vi "test controller.vi"() -> ()   [LabVIEW 2024, in "Lock-in module.lvlib"]
uses:
  Lock-in module.lvlib
  Messenger service/MessengerLib.lvlib
  Messenger service/Data types/Mailbox address.ctl
  ctl/MFLI_command enum.ctl
  ctl/MFLI_message for module.ctl
  <instrlib>/Zurich Instruments LabOne/Public/ziTypeHandle.ctl
  <instrlib>/Zurich Instruments LabOne/Zurich Instruments LabOne.lvlib
  <instrlib>/Zurich Instruments LabOne/Public/Data/ziTypeDemodSampleSingle.ctl
  ctl/MFLI parameters.ctl
  ctl/Mode.ctl
  ctl/ACQ info.ctl
panel:
  out "error out":errorcluster
  out "ignored error":errorcluster
  out "data":errorcluster
  out "Waveform Graph 3":dbl[](graph)
  out "LockIn info":T1
  out "data 2":T2={"Timestamps (ticks)"=0, "X (Vrms)"=nan, "Y (Vrms)"=nan, "Osc Phase (deg)"=nan, "Freq (Hz)"=nan, "DIO"=0, "AuxIn0 (V)"=nan, "AuxIn1 (V)"=nan, "Trigger"=0}
  out "Lock-in handle":T3 {"Handle" format="0x%08x"; "Conn" format="0x%08x"}
  out "Parameters out":T4={"Filter order"=1.0, "Time constant [ms]"=1.0, "F_Mod [kHz]"=0.0, "Amp_Mod [mV]"=0.0, "Enable output"=0, "Phase [°]"=0.0} {"Enable output" items=["Disable", "Enable"]; "Filter order" min=1.0 step=1.0; "Time constant [ms]" min=1.0 max=9.0 step=1.0}
  out "Array":string[](array[string])
  out "Connected device":string
  in  "Device name":string="DEV4029"
  in  "ACQ parameters":T4={"Filter order"=1.0, "Time constant [ms]"=1.0, "F_Mod [kHz]"=0.0, "Amp_Mod [mV]"=0.0, "Enable output"=0, "Phase [°]"=0.0} {"Enable output" items=["Disable", "Enable"]; "F_Mod [kHz]" min=0.1 max=100.0; "Filter order" min=1.0 max=9.0 step=1.0; "Time constant [ms]" min=0.001 max=1000000000.0}
  in  "Stop Button":bool
  in  "Connect":bool
  in  "Update settings":bool
  in  "Record":bool
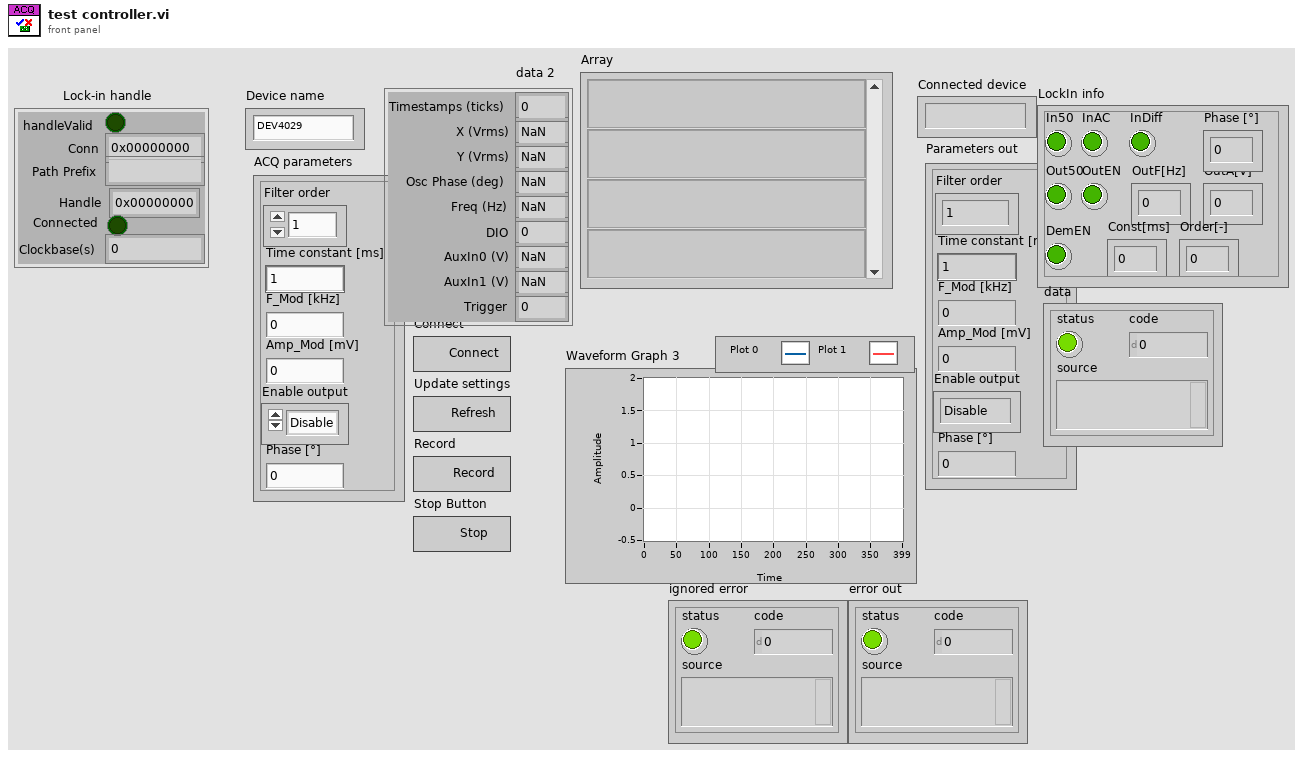
[diagram p1: front panel]
types:
  T1 = typedef "Lock-in module.lvlib/ACQ info.ctl" = cluster{"In50":bool, "InAC":bool, "InDiff":bool, "Out50":bool, "OutEN":bool, "OutF[Hz]":dbl, "OutA[V]":dbl, "DemEN":bool, "Const[ms]":dbl, "Order[-]":i32, "Phase [°]":dbl}
  T2 = typedef "Zurich Instruments LabOne.lvlib/ziTypeDemodSampleSingle.ctl" = cluster{"Timestamps (ticks)":u64, "X (Vrms)":dbl, "Y (Vrms)":dbl, "Osc Phase (deg)":dbl, "Freq (Hz)":dbl, "DIO":u32, "AuxIn0 (V)":dbl, "AuxIn1 (V)":dbl, "Trigger":u32}
  T3 = typedef "Zurich Instruments LabOne.lvlib/ziTypeHandle.ctl" = cluster{"handleValid":bool, "Conn":u64, "Path Prefix":string, "Handle":u64, "Connected":bool, "Clockbase(s)":dbl}
  T4 = typedef "Lock-in module.lvlib/MFLI parameters.ctl" = cluster{"Filter order":dbl, "Time constant [ms]":dbl, "F_Mod [kHz]":dbl, "Amp_Mod [mV]":dbl, "Enable output":u16, "Phase [°]":dbl}
  T5 = typedef "MessengerLib.lvlib/Mailbox address.ctl" = refnum<queue>
  T6 = typedef "MessengerLib.lvlib/Messenger referencies.ctl" = cluster{"TOP":refnum<queue>, "Instr_M":refnum<queue>, "Field_C":refnum<queue>, "Tmp_M":refnum<queue>, "Tmp_C":refnum<queue>, "Table_C":refnum<queue>, "MW_C":refnum<queue>, "Data_Aq":refnum<queue>, "Mod_M":refnum<queue>, "Field_M":refnum<queue>, "Pwr_M":refnum<queue>, "Angle_C":refnum<queue>, "Sample_C":refnum<queue>, "Reserved":refnum<queue>}
  T7 = typedef "Lock-in module.lvlib/MFLI_message for module.ctl" = cluster{"Command":T8, "Data":variant}
  T8 = typedef "Lock-in module.lvlib/MFLI_command enum.ctl" = enum16{"Initialize", "Update", "Set parameters", "Set module", "Set individual parameters", "Get point", "Get array", "Disconnect", "End", "Ignore"}
  T9 = typedef "Lock-in module.lvlib/Mode.ctl" = enum16{"None", "Point", "Scope", "Both", "DAQ"}
  T10 = typedef "MessengerLib.lvlib/MSG to TOP.ctl" = cluster{"Module":T11, "Response":string, "Data":variant, "Time":timestamp}
  T11 = typedef "Module name.ctl" = enum16{"Emty", "Magnet", "VTI", "Excitation", "Servo", "Acquisition", "Rotator", "Digitizer", "SMU2450", "Carousel", "Multimeter", "Tmp monitor", "Power monitor"}
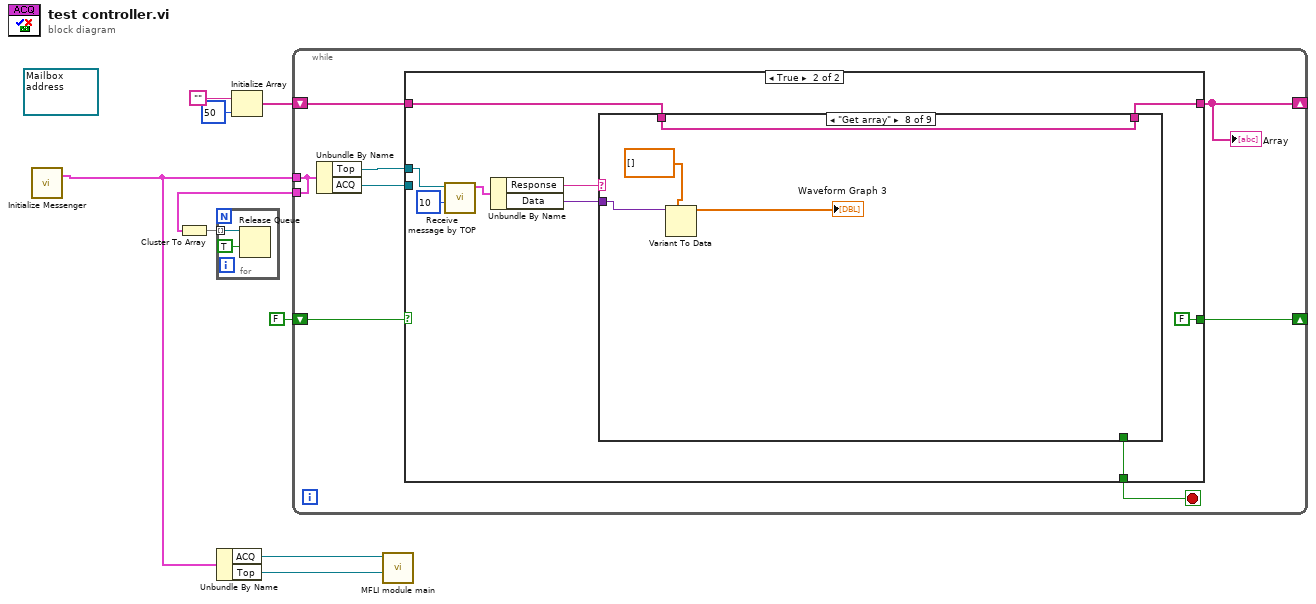
[diagram p0: block diagram]
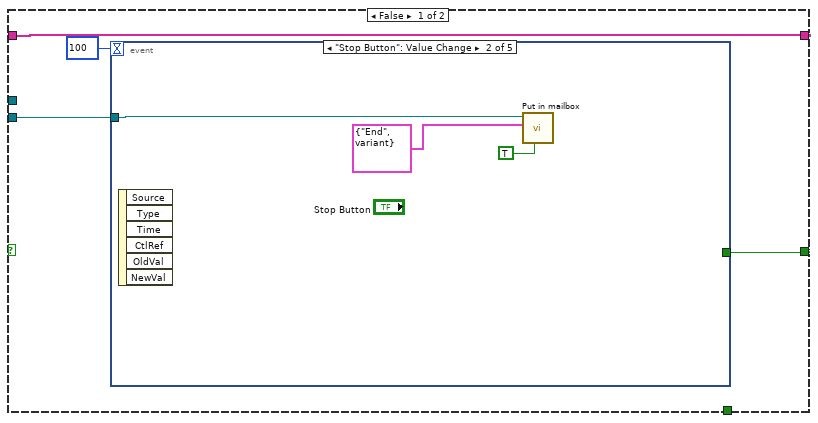
[diagram p2: hidden frame]
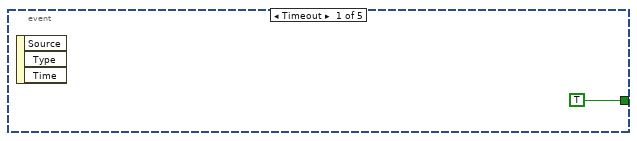
[diagram p3: hidden frame]
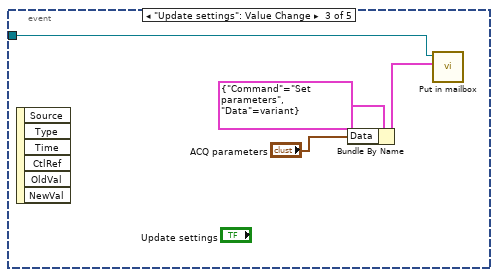
[diagram p4: hidden frame]
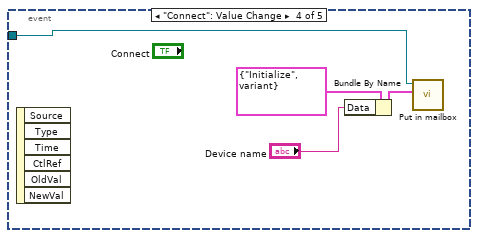
[diagram p5: hidden frame]
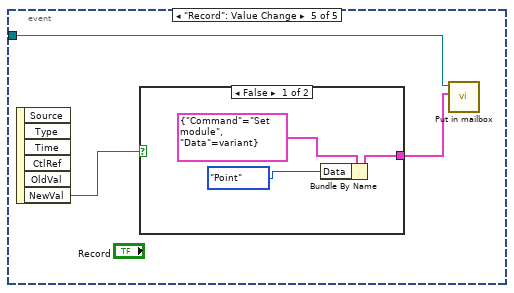
[diagram p6: hidden frame]
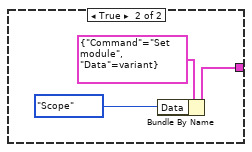
[diagram p7: hidden frame]
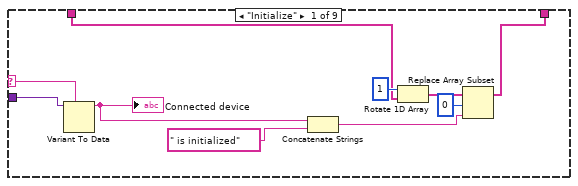
[diagram p8: hidden frame]
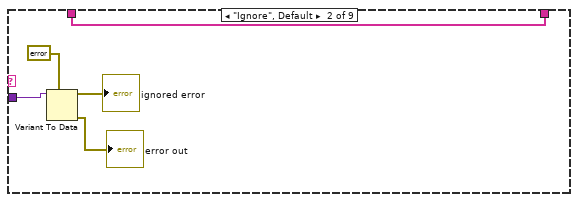
[diagram p9: hidden frame]
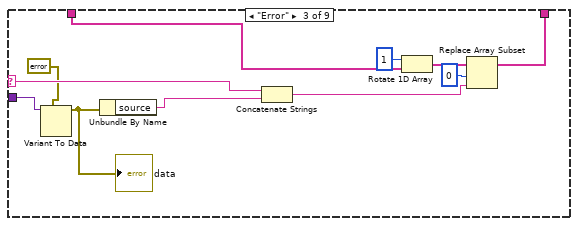
[diagram p10: hidden frame]
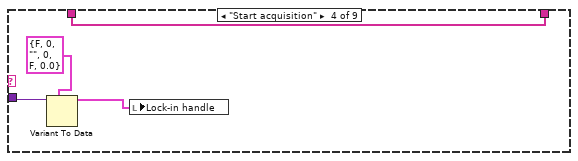
[diagram p11: hidden frame]
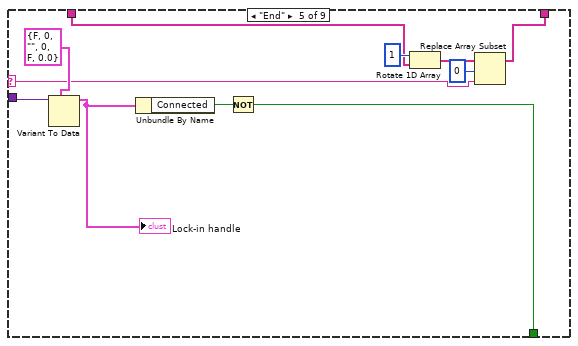
[diagram p12: hidden frame]
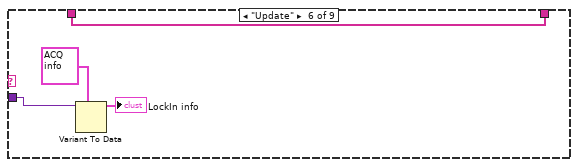
[diagram p13: hidden frame]
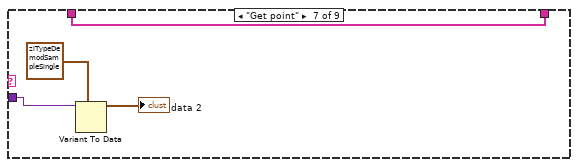
[diagram p14: hidden frame]
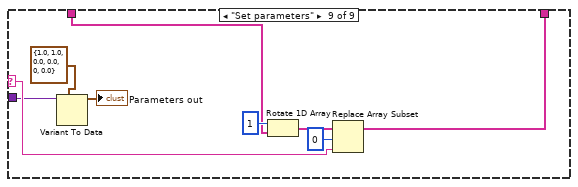
[diagram p15: hidden frame]
diagram:
  (unwired) T5 refnum ("Digitizer")
  n1 = call "Initialize Messenger.vi"() -> ("Referencies out"=w3:T6)  [unwired: 2 in, 1 out]
  n2 = Unbundle By Name(w3) -> ("ACQ"=w1:refnum<queue>, "Top"=w2:refnum<queue>)
  n3 = Initialize Array("", 50 ("dimension size")) -> (w4:string[])
  n4 = while {
    shift-right: [w16] -> _
    shift-left: FALSE -> [w17]
    tunnel: w3 -> [w12]
    tunnel: [w12] -> w8
    shift-right: [w10] -> _
    shift-left: w4 -> [w11]
    stop <- w15 stop-if-true
    n5 = Unbundle By Name(w12) -> ("Top"=w14:refnum<queue>, "ACQ"=w13:refnum<queue>)
    n6 = case shown="True" w17 {
      tunnel: [w20 FALSE] -> w16
      tunnel: w14 -> [_ w50]
      tunnel: w13 -> [w19 _]
      tunnel: [_ w46] -> w15
      tunnel: w11 -> [w18 w45]
      tunnel: [w18 w44] -> w10
      frame False {
        n7 = event shown="[1] \"Stop Button\": Value Change" {
          selector: _ -> [_ _ _ _ _]
          dyn-events: _ -> [_ _ _ _ _]
          timeout: 100 -> [_ _ _ _ _]
          tunnel: [TRUE _ _ _ _] -> w20
          tunnel: w19 -> [_ w25 w26 w32 w36]
          event Timeout {
            n8 = event-data() -> ()  [unwired: 1 in, 3 out]
          }
          event "Stop Button": Value Change {
            n9 = event-data() -> ()  [unwired: 1 in, 6 out]
            n10 = call "Put in mailbox.vi"("Priority? (F)"=TRUE, "Message"=T7 {"Command"=enum."End", "Data"=variant} ("MSG for  ACQ"), "Queue in"=w25) -> ()  [unwired: 6 in, 3 out]
          }
          event "Update settings": Value Change {
            n11 = event-data() -> ()  [unwired: 1 in, 6 out]
            n12 = Bundle By Name(cluster=T7 {"Command"=enum."Set parameters", "Data"=variant} ("MSG for  ACQ"), "Data"="ACQ parameters") -> (w28:T7)
            n13 = call "Put in mailbox.vi"("Message"=w28, "Queue in"=w26) -> ()  [unwired: 7 in, 3 out]
          }
          event "Connect": Value Change {
            n14 = event-data() -> ()  [unwired: 1 in, 6 out]
            n15 = Bundle By Name(cluster=T7 {"Command"=enum."Initialize", "Data"=variant} ("MSG for  ACQ"), "Data"="Device name") -> (w31:T7)
            n16 = call "Put in mailbox.vi"("Message"=w31, "Queue in"=w32) -> ()  [unwired: 7 in, 3 out]
          }
          event "Record": Value Change {
            n17 = event-data() -> ("NewVal"=w34:bool)  [unwired: 1 in, 5 out]
            n18 = case shown="False" w34 {
              tunnel: [w38 w41] -> w35
              frame False {
                n19 = Bundle By Name(cluster=T7 {"Command"=enum."Set module", "Data"=variant} ("MSG for  ACQ"), "Data"=Mode."Point" ("Mode")) -> (w38:T7)
              }
              frame True {
                n20 = Bundle By Name(cluster=T7 {"Command"=enum."Set module", "Data"=variant} ("MSG for  ACQ"), "Data"=Mode."Scope" ("Mode")) -> (w41:T7)
              }
            }
            n21 = call "Put in mailbox.vi"("Message"=w35, "Queue in"=w36) -> ()  [unwired: 7 in, 3 out]
          }
        }
      }
      frame True {
        n22 = call "Receive message by TOP.vi"("timeout (100)"=10 ("timeout (-1)"), "Mailbox in"=w50) -> ("MSG packet"=w49:T10)  [unwired: 6 in, 3 out]
        n23 = Unbundle By Name(w49) -> ("Response"=w48:string, "Data"=w47:variant)
        n24 = case shown="\"Get array\"" w48 {
          selector: w48 -> [w60 _ w73 _ w84 _ _ _ w108]
          tunnel: w47 -> [w61 w65 w71 w80 w92 w96 w100 w104 w107]
          tunnel: [_ _ _ _ w88 _ _ _ _] -> w46
          tunnel: w45 -> [w56 w66 w72 w81 w83 w95 w98 w103 w110]
          tunnel: [w55 w66 w74 w81 w82 w95 w98 w103 w109] -> w44
          frame "Initialize" {
            n25 = Variant To Data(type=w60, Variant=w61) -> (data=w54:string)  [unwired: 1 in, 1 out]
            "Connected device" <- w54
            n26 = Concatenate Strings(w54, " is initialized" ("string")) -> (w53:string)
            n27 = Rotate 1D Array(1:w56, 2:1 ("n")) -> (0:w59:string[])
            n28 = Replace Array Subset(array=w59, new element=w53, index=0) -> (w55:string[])
          }
          frame "Ignore", Default {
            n29 = Variant To Data(type=errorcluster {"status"=FALSE, "code"=0, "source"=""} ("error constant"), Variant=w65) -> (data=→"ignored error":errorcluster, error out=→"error out":errorcluster)  [unwired: 1 in]
          }
          frame "Error" {
            n30 = Variant To Data(type=errorcluster {"status"=FALSE, "code"=0, "source"=""} ("error constant"), Variant=w71) -> (data=w68:errorcluster)  [unwired: 1 in, 1 out]
            "data" <- w68
            n31 = Unbundle By Name(w68) -> ("source"=w67:string)
            n32 = Concatenate Strings(w73, w67) -> (w69:string)
            n33 = Rotate 1D Array(1:w72, 2:1 ("n")) -> (0:w77:string[])
            n34 = Replace Array Subset(array=w77, new element=w69, index=0) -> (w74:string[])
          }
          frame "Start acquisition" {
            n35 = Variant To Data(type=T3 {"handleValid"=FALSE, "Conn"=0, "Path Prefix"="", "Handle"=0, "Connected"=FALSE, "Clockbase(s)"=0.0} ("Lock-in Handle"), Variant=w80) -> (data=w78:T3)  [unwired: 1 in, 1 out]
            n36 = local write "Lock-in handle"(w78) -> ()
          }
          frame "End" {
            n37 = Variant To Data(type=T3 {"handleValid"=FALSE, "Conn"=0, "Path Prefix"="", "Handle"=0, "Connected"=FALSE, "Clockbase(s)"=0.0} ("Lock-in Handle"), Variant=w92) -> (data=w90:T3)  [unwired: 1 in, 1 out]
            "Lock-in handle" <- w90
            n38 = Unbundle By Name(w90) -> ("Connected"=w89:bool)
            n39 = Not(x=w89) -> (.not. x?=w88:bool)
            n40 = Rotate 1D Array(1:w83, 2:1 ("n")) -> (0:w87:string[])
            n41 = Replace Array Subset(array=w87, new element=w84, index=0) -> (w82:string[])
          }
          frame "Update" {
            n42 = Variant To Data(type=T1 {"In50"=FALSE, "InAC"=FALSE, "InDiff"=FALSE, "Out50"=FALSE, "OutEN"=FALSE, "OutF[Hz]"=0.0, "OutA[V]"=0.0, "DemEN"=FALSE, "Const[ms]"=0.0, "Order[-]"=0, "Phase [°]"=0.0} ("Cluster"), Variant=w96) -> (data=→"LockIn info":T1)  [unwired: 1 in, 1 out]
          }
          frame "Get point" {
            n43 = Variant To Data(type=T2 {"Timestamps (ticks)"=0, "X (Vrms)"=nan, "Y (Vrms)"=nan, "Osc Phase (deg)"=nan, "Freq (Hz)"=nan, "DIO"=0, "AuxIn0 (V)"=nan, "AuxIn1 (V)"=nan, "Trigger"=0} ("Demod Sample Out"), Variant=w100) -> (data=→"data 2":T2)  [unwired: 1 in, 1 out]
          }
          frame "Get array" {
            n44 = Variant To Data(type=dbl[] [], Variant=w104) -> (data=→"Waveform Graph 3":dbl[])  [unwired: 1 in, 1 out]
          }
          frame "Set parameters" {
            n45 = Variant To Data(type=T4 {"Filter order"=1.0, "Time constant [ms]"=1.0, "F_Mod [kHz]"=0.0, "Amp_Mod [mV]"=0.0, "Enable output"=0, "Phase [°]"=0.0} ("ACQ parameters"), Variant=w107) -> (data=→"Parameters out":T4)  [unwired: 1 in, 1 out]
            n46 = Rotate 1D Array(1:w110, 2:1 ("n")) -> (0:w113:string[])
            n47 = Replace Array Subset(array=w113, new element=w108, index=0) -> (w109:string[])
          }
        }
      }
    }
    "Array" <- w10
  }
  n48 = Cluster To Array(cluster=w8) -> (array=w7:refnum<queue>[])
  n49 = for {
    tunnel: w7 -> [w115] mode=indexing
    n50 = Release Queue(queue=w115, force destroy? (F)=TRUE) -> ()  [unwired: 1 in, 3 out]
  }
  n51 = call "MFLI module main.vi"("Master mailbox"=w2, "Module mailbox"=w1) -> ()  [unwired: 10 in]
